vi "Send Run VI.vi"(4 "Open Front Panel":bool, 5 "Indicator Names":string[](array[string]), 6 "Run Options":i32, 7 "Message Priority (Normal)":T1=enum."Normal", 8 "error in (no error)":errorcluster, 9 "VI Control Values":refnum<class "tBSONDocument.lvclass">, 10 "VI Path":string, 11 "Message Enqueuer":refnum<class "Message Enqueuer.lvclass">) -> (0 "error out":errorcluster, 3 "Message Enqueuer out":refnum<class "Message Enqueuer.lvclass">)   [LabVIEW 2014, in "tWorkerCommandRunner.lvlib" / "Run VI.lvclass"]
doc: "This VI sends the message to an actor."
uses:
  Run VI.lvclass
  <vilib>/ActorFramework/Message Enqueuer/Message Enqueuer.lvclass
  <vilib>/ActorFramework/Message Enqueuer/Message Priority.ctl
  BSON/tBSONDocument/tBSONDocument.lvclass
  Run VI.lvclass/Run VI.ctl
  <vilib>/ActorFramework/Message Enqueuer/Message Enqueuer.lvclass/Message Enqueuer.ctl
  <vilib>/ActorFramework/Message Priority Queue/Priority Enqueue.vi
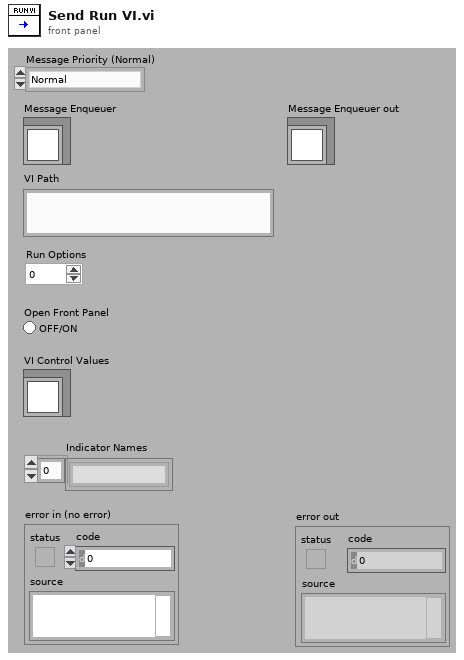
[diagram p1: front panel]
types:
  T1 = typedef "Actor Framework.lvlib/Message Enqueuer.lvclass/Message Priority.ctl" = enum16{"Low", "Normal", "High"}
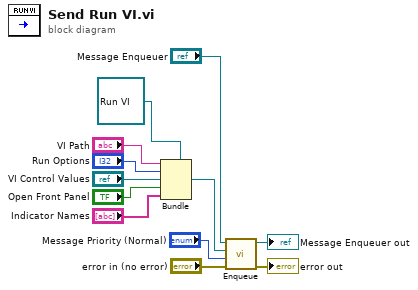
[diagram p0: block diagram]
diagram:
  n1 = Bundle(cluster=refnum<class "Run VI.lvclass"> refnum ("Object"), "VI Path", "Run Options", "VI Control Values", "Open Front Panel", "Indicator Names") -> (w8:refnum<class "Run VI.lvclass">)
  n2 = call <vilib>:"Enqueue.vi"("error in (no error)"="error in (no error)", "Message Priority (Normal)"="Message Priority (Normal)", "Message"=w8, "Message Enqueuer in"="Message Enqueuer") -> ("error out"=→"error out":errorcluster, "Message Enqueuer out"=→"Message Enqueuer out":refnum<class "Message Enqueuer.lvclass">)  [unwired: 6 in]
